vi "fuzzyex Animate Rotating Wheel.vi"(8 "Angle (deg)":dbl format="%.2f") -> (3 "new picture":picture)   [LabVIEW 2023]
doc: "This VI draws the steering wheel based on the input Angle."
uses:
  <vilib>/picture/picture.llb/imagedata.ctl
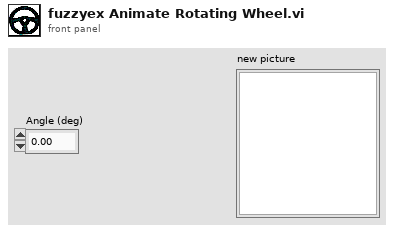
[diagram p1: front panel]
types:
  T1 = typedef "imagedata.ctl" = cluster{"image type":i32, "image depth":i32, "image":u8[], "mask":u8[], "colors":u32[], "Rectangle":cluster{"left":i16, "top":i16, "right":i16, "bottom":i16}}
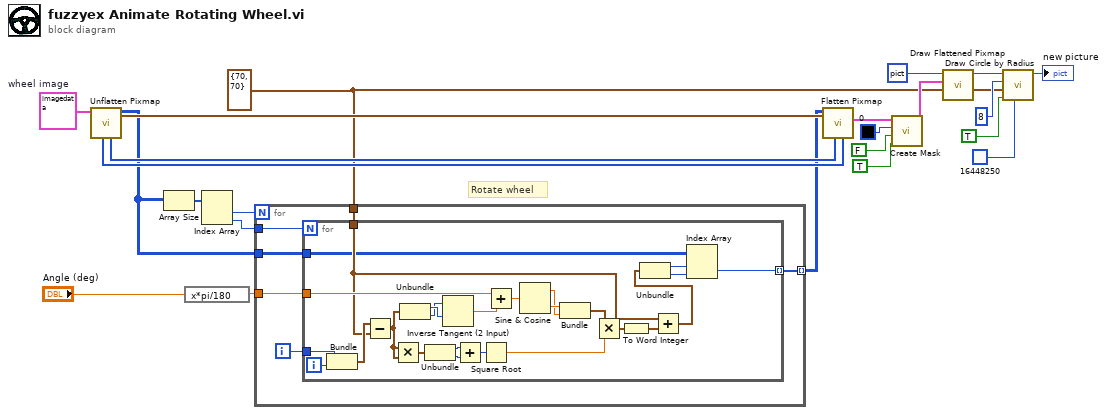
[diagram p0: block diagram]
diagram:
  w20 = T1 {"image type"=0, "image depth"=24, "image"=array[58800 elements], "mask"=[], "colors"=[], "Rectangle"={"left"=0, "top"=0, "right"=140, "bottom"=140}}  # wheel image
  w3 = cluster{"x":i16, "y":i16} {"x"=70, "y"=70} ("Center 2")
  # "Rotate wheel"
  n1 = call <vilib>:"Unflatten Pixmap.vi"("image data"=w20) -> ("24-bit pixmap"=w2:u32[][], "colors"=w18:u32[], "top left"=w19:cluster{"x":i16, "y":i16}, "mask"=w10:u8[])  [unwired: 7 out]
  n2 = Array Size(array=w2) -> (size(s)=w23:i32[])
  n3 = expression code="x*pi/180"("Angle (deg)") -> (w6:dbl)
  n4 = Index Array(array=w23) -> (element #1=w21:i32, element #2=w22:i32)  [unwired: 2 in]
  n5 = for {
    N: w21 -> [_]
    tunnel: w22 -> [w29]
    tunnel: w6 -> [w28]
    tunnel: w3 -> [w27]
    tunnel: w2 -> [w25]
    tunnel: [w24] -> w1 mode=indexing
    i -> [w26]
    n6 = for {
      N: w29 -> [_]
      tunnel: w26 -> [w54]
      tunnel: w28 -> [w44]
      tunnel: w27 -> [w33]
      tunnel: w25 -> [w31]
      tunnel: [w30] -> w24 mode=indexing
      i -> [w32]
      n7 = Bundle(w54, w32) -> (w53:cluster{i32, i32})  [unwired: 1 out]
      n8 = Subtract(x=w53, y=w33) -> (x-y=w48:cluster{i32, i32})
      n9 = Multiply(x=w48, y=w48) -> (x*y=w52:cluster{i32, i32})
      n10 = Unbundle(w48) -> (w47:i32, w46:i32)
      n11 = Unbundle(w52) -> (w51:i32, w50:i32)
      n12 = Inverse Tangent (2 Input)(1:w47, 2:w46) -> (0:w45:dbl)
      n13 = Add(x=w51, y=w50) -> (x+y=w49:i32)
      n14 = Square Root(x=w49) -> (sqrt(x)=w39:dbl)
      n15 = Add(x=w44, y=w45) -> (x+y=w43:dbl)
      n16 = Sine & Cosine(0:w43) -> (1:w41:dbl, 2:w42:dbl)
      n17 = Bundle(w42, w41) -> (w40:cluster{dbl, dbl})  [unwired: 1 out]
      n18 = Multiply(x=w40, y=w39) -> (x*y=w38:cluster{dbl, dbl})
      n19 = To Word Integer(number=w38) -> (16bit integer=w37:cluster{i16, i16})
      n20 = Add(x=w33, y=w37) -> (x+y=w34:cluster{i16, i16})
      n21 = Unbundle(w34) -> (w36:i16, w35:i16)
      n22 = Index Array(array=w31, index (row)=w36, index (col)=w35) -> (element=w30:u32)
    }
  }
  n23 = call <vilib>:"Flatten Pixmap.vi"("mask"=w10, "colors"=w18, "top left"=w19, "24-bit pixmap"=w1) -> ("image data"=w12:T1)  [unwired: 3 in, 4 out]
  n24 = call <vilib>:"Create Mask.vi"("Combine Masks? (F)"=TRUE, "1-Bit Mask Value (T)"=FALSE, "Mask Color (Black)"=u32 0, "image data"=w12) -> ("image data"=w11:T1)  [unwired: 7 out]
  n25 = call <vilib>:"Draw Flattened Pixmap.vi"("image data"=w11, "picture"=picture data[5B]) -> ("new picture"=w17:picture)  [unwired: 7 out]
  n26 = call <vilib>:"Draw Circle by Radius.vi"("color(black)"=u32 16448250, "fill?(F)"=TRUE, "pixel center"=w3, "radius"=i16 8, "picture"=w17) -> ("new picture"=→"new picture":picture)  [unwired: 3 in, 3 out]
